vi "HAL camera set temp.vi"(1 "Temp. Set Point":i32) -> (0 "error out":errorcluster)   [LabVIEW 2011]
uses:
  Cascade-specific globals.vi
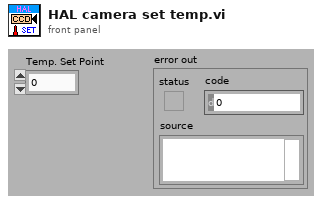
[diagram p1: front panel]
types:
  T1 = cluster{"Camera Handle":u32, "Pulser Handle":u32, "File Handle":u32, "Display Handle":u32, "Image Handle":u32}
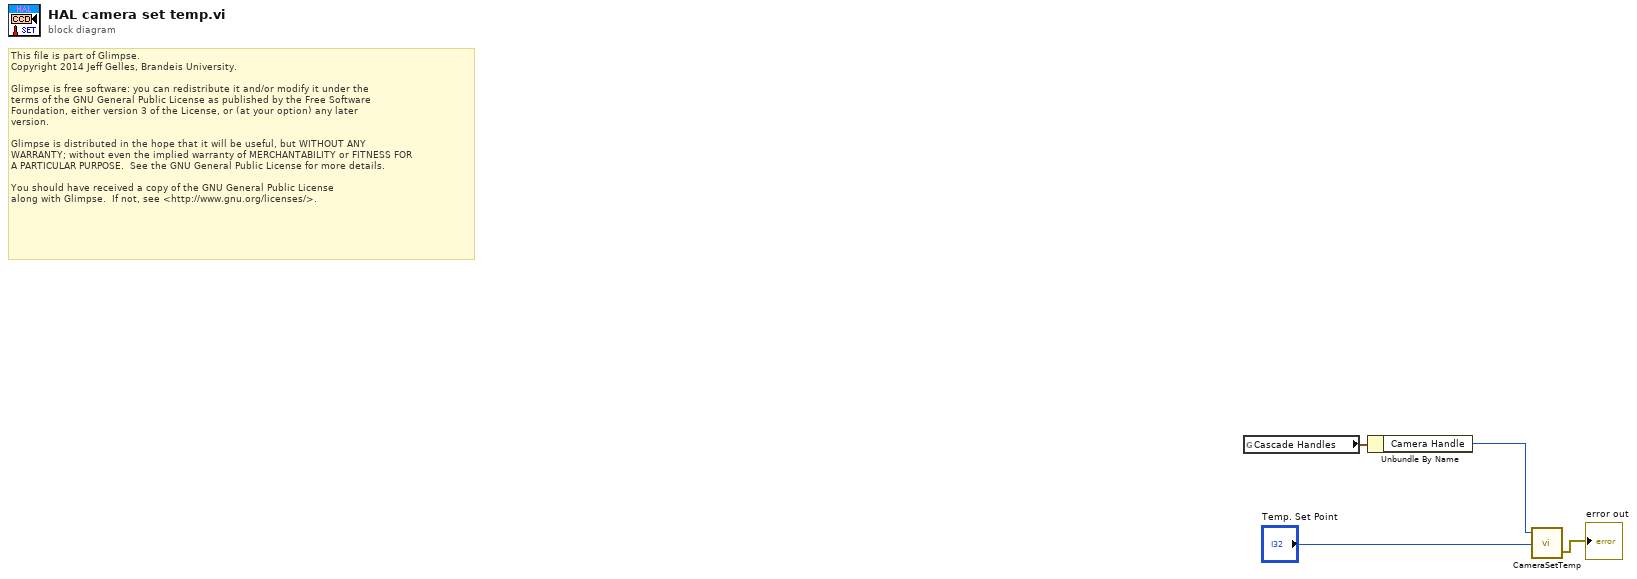
[diagram p0: block diagram]
diagram:
  # "This file is part of Glimpse. \nCopyright 2014 Jeff Gelles, Brandeis University.    \n\nGlimpse is free software: you can redistribute it and/or modify it under the \nterms of the GNU General Public License as published by the Free Software \nFoundation, either version 3 of the License, or (at your option) any later \nversion.\n\nGlimpse is distributed in the hope that it will be useful, but WITHOUT ANY \nWARRANTY; without even the implied warranty of MERCHANTABILITY or FITNESS FOR \nA PARTICULAR PURPOSE.  See the GNU General Public License for more details.\n\nYou should have received a copy of the GNU General Public License\nalong with Glimpse.  If not, see <http://www.gnu.org/licenses/>."
  n1 = global read "Cascade-specific globals.vi" "Cascade Handles"() -> (w2:T1)
  n2 = Unbundle By Name(w2) -> ("Camera Handle"=w1:u32)
  n3 = call <userlib>:"CameraSetTemp.vi"("Temperature"="Temp. Set Point", "Camera Handle"=w1) -> ("error out"=→"error out":errorcluster)  [unwired: 1 in, 1 out]
